vi "Clusters.vi"() -> ()   [LabVIEW 2018]
panel:
  out "Comparison Result":T1
  in  "Input Cluster 2":T2
  in  "Input Cluster 1":T2
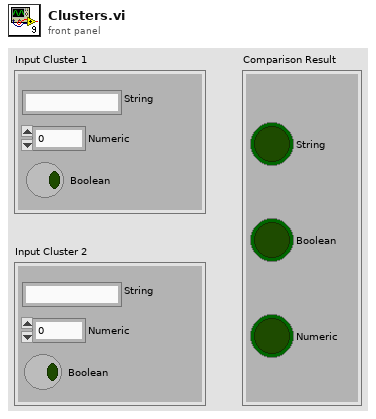
[diagram p1: front panel]
types:
  T1 = cluster{"String":bool, "Boolean":bool, "Numeric":bool}
  T2 = cluster{"String":string, "Boolean":bool, "Numeric":dbl}
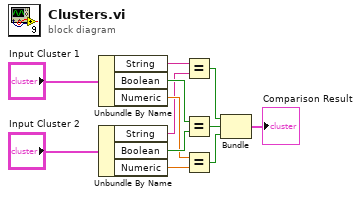
[diagram p0: block diagram]
diagram:
  n1 = Unbundle By Name("Input Cluster 1") -> ("String"=w3:string, "Boolean"=w10:bool, "Numeric"=w7:dbl)
  n2 = Unbundle By Name("Input Cluster 2") -> ("String"=w2:string, "Boolean"=w9:bool, "Numeric"=w8:dbl)
  n3 = Equal?(x=w3, y=w2) -> (x = y?=w1:bool)
  n4 = Equal?(x=w10, y=w9) -> (x = y?=w5:bool)
  n5 = Equal?(x=w7, y=w8) -> (x = y?=w4:bool)
  n6 = Bundle(w1, w5, w4) -> (→"Comparison Result":cluster{bool, bool, bool})  [unwired: 1 in]
